vi "LMS_GetSampleRate.vi"(8 "error in (no error)":errorcluster, 9 "chan":u64, 10 "dir_tx":u8, 11 "device_In":i64) -> (0 "error out":errorcluster, 1 "host_exchange Rage Hz":dbl, 3 "device_Out":i64, 4 "RF_Hz":dbl)   [LabVIEW 2018, in "LMS_LV_Drv.lvlib"]
uses:
  LMS_LV_Drv.lvlib
  C:/Program Files/PothosSDR/bin/LimeSuite.dll
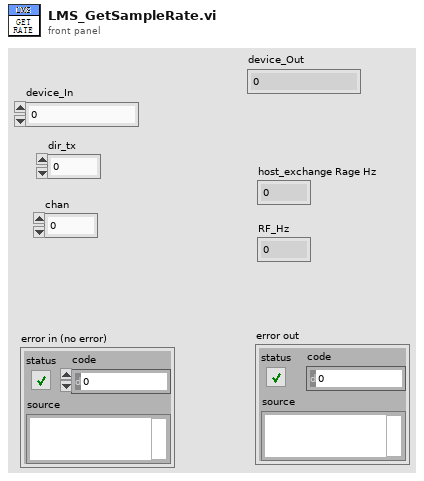
[diagram p1: front panel]
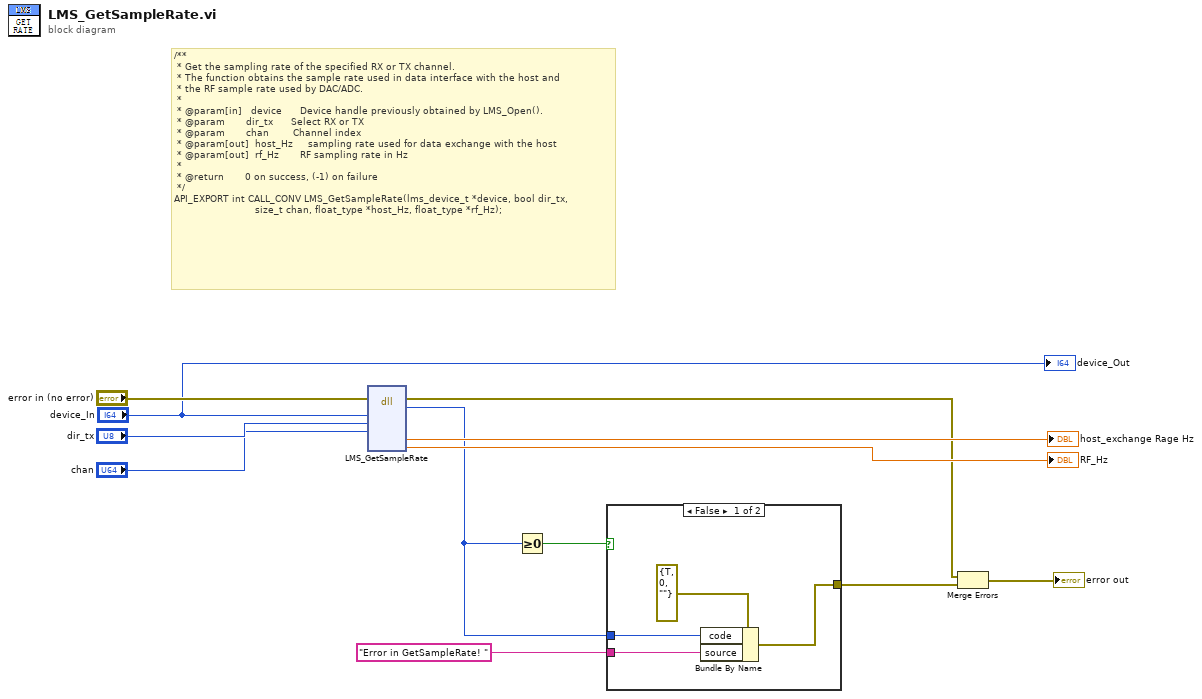
[diagram p0: block diagram]
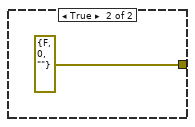
[diagram p2: hidden frame]
diagram:
  # "/**\n * Get the sampling rate of the specified RX or TX channel.\n * The function obtains the sample rate used in data interface with the host and\n * the RF sample rate used by DAC/ADC.\n *\n * @param[in]   device      Device handle previously obtained by LMS_Open().\n * @param       dir_tx      Select RX or TX\n * @param       chan        Channel index\n * @param[out]  host_Hz     sampling rate used for data exchange with the host\n * @param[out]  rf_Hz       RF sampling rate in Hz\n *\n * @return       0 on success, (-1) on failure\n */\nAPI_EXPORT int CALL_CONV LMS_GetSampleRate(lms_device_t *device, bool dir_tx,\n                           size_t chan, float_type *host_Hz, float_type *rf_Hz);"
  n1 = dll-call lib="C:/Program Files/PothosSDR/bin/LimeSuite.dll" fn="LMS_GetSampleRate"(error in="error in (no error)", "device"="device_In", "dir_tx"="dir_tx", "chan"="chan") -> (error out=w2:errorcluster, "return type"=w3:i32, "host_Hz"=→"host_exchange Rage Hz":dbl, "rf_Hz"=→"RF_Hz":dbl)  [unwired: 7 in, 1 out]
  n2 = Greater Or Equal To 0?(x=w3) -> (x >= 0?=w6:bool)
  n3 = case shown="False" w6 {
    tunnel: [w15 errorcluster {"status"=FALSE, "code"=0, "source"=""} ("error in")] -> w4
    tunnel: w3 -> [w14 _]
    tunnel: "Error in GetSampleRate! " ("source") -> [w13 _]
    frame False {
      n4 = Bundle By Name(cluster=errorcluster {"status"=TRUE, "code"=0, "source"=""} ("error in"), "code"=w14, "source"=w13) -> (w15:errorcluster)
    }
    frame True {
    }
  }
  n5 = Merge Errors(w2, w4) -> (→"error out":errorcluster)
  "device_Out" <- "device_In"
